vi "LV Demo Main.vi"() -> ()   [LabVIEW 2018, in "Powermeter_library.lvlib"]
uses:
  Powermeter_library.lvlib
  Channel States.ctl
  Global Variables.vi
  <vilib>/regexp/Match Regular Expression.xnode
panel:
  out "tdms error":errorcluster
  out "tdms file":refnum<k34>
  out "File Size (Mb)":dbl=76.0
  in  "Tab Control":enum32{"File", "Page 2"}(tab)
  out "file path":path=path "E:/Alkali metals/Excimer/2018-03-05/Run1_Powermeter.tdms"
  in  "Logfile?":bool=TRUE
  in  "Meas On":bool[](array[boolean])=[FALSE]
  in  "scan again":bool
  in  "All Handles":i32[](array[numeric])=[0]
  in  "Get Lib Ver":bool
  in  "Get Driver Ver":bool
  out "LibVer":i32
  out "DriverVer":string
  out "output cluster":T1
  in  "Reset graph 2":bool
  out "Timestamp offset":dbl
  out "First Data point":bool=TRUE
  out "Power meter 2":cluster{timestamp[], dbl[]}(graph)={[timestamp(3586444920.089349 s since 1904-01-01), timestamp(3586444920.2053604 s since 1904-01-01), timestamp(3586444920.2613664 s since 1904-01-01), timestamp(3586444920.370377 s since 1904-01-01), timestamp(3586444920.479388 s since 1904-01-01), timestamp(3586444920.588399 s since 1904-01-01), timestamp(3586444920.70241 s since 1904-01-01), timestamp(3586444920.7584157 s since 1904-01-01), timestamp(3586444920.868427 s since 1904-01-01), timestamp(3586444920.978438 s since 1904-01-01), timestamp(3586444921.0864487 s since 1904-01-01), timestamp(3586444921.19646 s since 1904-01-01), timestamp(3586444921.253465 s since 1904-01-01), timestamp(3586444921.3664765 s since 1904-01-01), timestamp(3586444921.6875086 s since 1904-01-01), timestamp(3586444921.7935195 s since 1904-01-01), timestamp(3586444922.0625463 s since 1904-01-01), timestamp(3586444922.170557 s since 1904-01-01), timestamp(3586444922.491589 s since 1904-01-01), timestamp(3586444922.6016 s since 1904-01-01), timestamp(3586444922.868627 s since 1904-01-01), timestamp(3586444922.977638 s since 1904-01-01), timestamp(3586444923.29867 s since 1904-01-01), timestamp(3586444923.3546753 s since 1904-01-01), timestamp(3586444923.6767077 s since 1904-01-01), timestamp(3586444923.7857184 s since 1904-01-01), timestamp(3586444924.0537453 s since 1904-01-01), timestamp(3586444924.161756 s since 1904-01-01), timestamp(3586444924.270767 s since 1904-01-01), timestamp(3586444924.379778 s since 1904-01-01), timestamp(3586444924.489789 s since 1904-01-01), timestamp(3586444924.6028004 s since 1904-01-01), timestamp(3586444924.6558056 s since 1904-01-01), timestamp(3586444924.772817 s since 1904-01-01), timestamp(3586444924.880828 s since 1904-01-01), timestamp(3586444924.952835 s since 1904-01-01), timestamp(3586444925.062846 s since 1904-01-01), timestamp(3586444925.168857 s since 1904-01-01), timestamp(3586444925.2788677 s since 1904-01-01), timestamp(3586444925.3868785 s since 1904-01-01), timestamp(3586444925.4968896 s since 1904-01-01), timestamp(3586444925.552895 s since 1904-01-01), timestamp(3586444925.6619062 s since 1904-01-01), timestamp(3586444925.770917 s since 1904-01-01), timestamp(3586444925.879928 s since 1904-01-01), timestamp(3586444925.987939 s since 1904-01-01), timestamp(3586444926.0939493 s since 1904-01-01), timestamp(3586444926.149955 s since 1904-01-01), timestamp(3586444926.2609663 s since 1904-01-01), timestamp(3586444926.370977 s since 1904-01-01), timestamp(3586444926.479988 s since 1904-01-01), timestamp(3586444926.588999 s since 1904-01-01), timestamp(3586444926.69801 s since 1904-01-01), timestamp(3586444926.7540154 s since 1904-01-01), timestamp(3586444926.863026 s since 1904-01-01), timestamp(3586444926.9760375 s since 1904-01-01), timestamp(3586444927.0850487 s since 1904-01-01), timestamp(3586444927.191059 s since 1904-01-01), timestamp(3586444927.30207 s since 1904-01-01), timestamp(3586444927.356076 s since 1904-01-01), timestamp(3586444927.4650865 s since 1904-01-01), timestamp(3586444927.5790977 s since 1904-01-01), timestamp(3586444927.688109 s since 1904-01-01), timestamp(3586444927.849125 s since 1904-01-01), timestamp(3586444927.9581356 s since 1904-01-01), timestamp(3586444928.0681467 s since 1904-01-01), timestamp(3586444928.180158 s since 1904-01-01), timestamp(3586444928.289169 s since 1904-01-01), timestamp(3586444928.39818 s since 1904-01-01), timestamp(3586444928.4661865 s since 1904-01-01), timestamp(3586444928.581198 s since 1904-01-01), timestamp(3586444928.6942096 s since 1904-01-01), timestamp(3586444928.750215 s since 1904-01-01), timestamp(3586444928.870227 s since 1904-01-01), timestamp(3586444928.9772377 s since 1904-01-01), timestamp(3586444929.0932493 s since 1904-01-01), timestamp(3586444929.149255 s since 1904-01-01), timestamp(3586444929.259266 s since 1904-01-01), timestamp(3586444929.3672767 s since 1904-01-01), timestamp(3586444929.4762874 s since 1904-01-01), timestamp(3586444929.5852985 s since 1904-01-01), timestamp(3586444929.694309 s since 1904-01-01), timestamp(3586444929.750315 s since 1904-01-01), timestamp(3586444929.862326 s since 1904-01-01), timestamp(3586444929.9763374 s since 1904-01-01), timestamp(3586444930.0863485 s since 1904-01-01), timestamp(3586444930.1943593 s since 1904-01-01), timestamp(3586444930.249365 s since 1904-01-01), timestamp(3586444930.358376 s since 1904-01-01), timestamp(3586444930.4763875 s since 1904-01-01), timestamp(3586444930.5853987 s since 1904-01-01), timestamp(3586444930.6944094 s since 1904-01-01), timestamp(3586444930.7514153 s since 1904-01-01), timestamp(3586444930.859426 s since 1904-01-01), timestamp(3586444930.9654365 s since 1904-01-01), timestamp(3586444931.0754476 s since 1904-01-01), timestamp(3586444931.190459 s since 1904-01-01), timestamp(3586444931.29947 s since 1904-01-01), timestamp(3586444931.3554754 s since 1904-01-01), timestamp(3586444931.4644866 s since 1904-01-01), timestamp(3586444931.7845182 s since 1904-01-01), timestamp(3586444931.8935294 s since 1904-01-01), timestamp(3586444931.949535 s since 1904-01-01), timestamp(3586444932.059546 s since 1904-01-01), timestamp(3586444932.1685567 s since 1904-01-01), timestamp(3586444932.277568 s since 1904-01-01), timestamp(3586444932.3875785 s since 1904-01-01), timestamp(3586444932.4965897 s since 1904-01-01), timestamp(3586444932.552595 s since 1904-01-01), timestamp(3586444932.6616063 s since 1904-01-01), timestamp(3586444932.770617 s since 1904-01-01), timestamp(3586444932.8796277 s since 1904-01-01), timestamp(3586444932.9866385 s since 1904-01-01), timestamp(3586444933.0956497 s since 1904-01-01), timestamp(3586444933.151655 s since 1904-01-01), timestamp(3586444933.2616663 s since 1904-01-01), timestamp(3586444933.374677 s since 1904-01-01), timestamp(3586444933.4836884 s since 1904-01-01), timestamp(3586444933.592699 s since 1904-01-01), timestamp(3586444933.649705 s since 1904-01-01), timestamp(3586444933.7587156 s since 1904-01-01), timestamp(3586444933.8667264 s since 1904-01-01), timestamp(3586444933.9757376 s since 1904-01-01), timestamp(3586444934.0837483 s since 1904-01-01), timestamp(3586444934.191759 s since 1904-01-01), timestamp(3586444934.29977 s since 1904-01-01), timestamp(3586444934.3557754 s since 1904-01-01), timestamp(3586444934.4647865 s since 1904-01-01), timestamp(3586444934.573797 s since 1904-01-01), timestamp(3586444934.6828084 s since 1904-01-01), timestamp(3586444934.791819 s since 1904-01-01), timestamp(3586444934.89883 s since 1904-01-01), timestamp(3586444934.9548354 s since 1904-01-01), timestamp(3586444935.063846 s since 1904-01-01), timestamp(3586444935.171857 s since 1904-01-01), timestamp(3586444935.280868 s since 1904-01-01), timestamp(3586444935.3898787 s since 1904-01-01), timestamp(3586444935.49989 s since 1904-01-01), timestamp(3586444935.5568957 s since 1904-01-01), timestamp(3586444935.6659064 s since 1904-01-01), timestamp(3586444935.770917 s since 1904-01-01), timestamp(3586444935.879928 s since 1904-01-01), timestamp(3586444935.988939 s since 1904-01-01), timestamp(3586444936.0979495 s since 1904-01-01), timestamp(3586444936.1539555 s since 1904-01-01), timestamp(3586444936.261966 s since 1904-01-01), timestamp(3586444936.370977 s since 1904-01-01), timestamp(3586444936.479988 s since 1904-01-01), timestamp(3586444936.588999 s since 1904-01-01), timestamp(3586444936.69901 s since 1904-01-01), timestamp(3586444936.7550154 s since 1904-01-01), timestamp(3586444936.864026 s since 1904-01-01), timestamp(3586444936.9720373 s since 1904-01-01), timestamp(3586444937.081048 s since 1904-01-01), timestamp(3586444937.189059 s since 1904-01-01), timestamp(3586444937.29907 s since 1904-01-01), timestamp(3586444937.3550754 s since 1904-01-01), timestamp(3586444937.4640865 s since 1904-01-01), timestamp(3586444937.573097 s since 1904-01-01), timestamp(3586444937.6831083 s since 1904-01-01)], [0.0, 0.0, 0.0, 0.0, 0.0, 0.0, 0.0, 0.0, 0.0, 0.0, 0.0, 0.0, 0.0, 0.0, 0.0, 0.0, 0.0, 0.0, 0.0, 0.0, 0.0, 0.0, 0.0, 0.0, 0.0, 0.0, 0.0, 0.0, 0.0, 0.0, 0.0, 0.0, 0.0, 0.0, 0.0, 0.0, 0.0, 0.0, 0.0, 0.0, 0.0, 0.0, 0.0, 0.0, 0.0, 0.0, 0.0, 0.0, 0.0, 0.0, 0.0, 0.0, 0.0, 0.0, 0.0, 0.0, 0.0, 0.0, 0.0, 0.0, 0.0, 0.0, 0.0, 0.0, 0.0, 0.0, 0.0, 0.0, 0.0, 0.0, 0.0, 0.0, 0.0, 0.0, 0.0, 0.0, 0.0, 0.0, 0.0, 0.0, 0.0, 0.0, 0.0, 0.0, 0.0, 0.0, 0.0, 0.0, 0.0, 0.0, 0.0, 0.0, 0.0, 0.0, 0.0, 0.0, 0.0, 0.0, 0.0, 0.0, 0.0, 0.0, 0.0, 0.0, 0.0, 0.0, 0.0, 0.0, 0.0, 0.0, 0.0, 0.0, 0.0, 0.0, 0.0, 0.0, 0.0, 0.0, 0.0, 0.0, 0.0, 0.0, 0.0, 0.0, 0.0, 0.0, 0.0, 0.0, 0.0, 0.0, 0.0, 0.0, 0.0, 0.0, 0.0, 0.0, 0.0, 0.0, 0.0, 0.0, 0.0, 0.0, 0.0, 0.0, 0.0, 0.0, 0.0, 0.0, 0.0, 0.0, 0.0, 0.0, 0.0, 0.0, 0.0, 0.0, 0.0, 0.0, 0.0, 0.0]}
  in  "Reset graph 1":bool
  out "Power meter 1":cluster{timestamp[], dbl[]}(graph)={[timestamp(3586444920.089349 s since 1904-01-01), timestamp(3586444920.2053604 s since 1904-01-01), timestamp(3586444920.2613664 s since 1904-01-01), timestamp(3586444920.370377 s since 1904-01-01), timestamp(3586444920.479388 s since 1904-01-01), timestamp(3586444920.588399 s since 1904-01-01), timestamp(3586444920.70241 s since 1904-01-01), timestamp(3586444920.7584157 s since 1904-01-01), timestamp(3586444920.868427 s since 1904-01-01), timestamp(3586444920.978438 s since 1904-01-01), timestamp(3586444921.0864487 s since 1904-01-01), timestamp(3586444921.19646 s since 1904-01-01), timestamp(3586444921.253465 s since 1904-01-01), timestamp(3586444921.3664765 s since 1904-01-01), timestamp(3586444921.6875086 s since 1904-01-01), timestamp(3586444921.7935195 s since 1904-01-01), timestamp(3586444922.0625463 s since 1904-01-01), timestamp(3586444922.170557 s since 1904-01-01), timestamp(3586444922.491589 s since 1904-01-01), timestamp(3586444922.6016 s since 1904-01-01), timestamp(3586444922.868627 s since 1904-01-01), timestamp(3586444922.977638 s since 1904-01-01), timestamp(3586444923.29867 s since 1904-01-01), timestamp(3586444923.3546753 s since 1904-01-01), timestamp(3586444923.6767077 s since 1904-01-01), timestamp(3586444923.7857184 s since 1904-01-01), timestamp(3586444924.0537453 s since 1904-01-01), timestamp(3586444924.161756 s since 1904-01-01), timestamp(3586444924.270767 s since 1904-01-01), timestamp(3586444924.379778 s since 1904-01-01), timestamp(3586444924.489789 s since 1904-01-01), timestamp(3586444924.6028004 s since 1904-01-01), timestamp(3586444924.6558056 s since 1904-01-01), timestamp(3586444924.772817 s since 1904-01-01), timestamp(3586444924.880828 s since 1904-01-01), timestamp(3586444924.952835 s since 1904-01-01), timestamp(3586444925.062846 s since 1904-01-01), timestamp(3586444925.168857 s since 1904-01-01), timestamp(3586444925.2788677 s since 1904-01-01), timestamp(3586444925.3868785 s since 1904-01-01), timestamp(3586444925.4968896 s since 1904-01-01), timestamp(3586444925.552895 s since 1904-01-01), timestamp(3586444925.6619062 s since 1904-01-01), timestamp(3586444925.770917 s since 1904-01-01), timestamp(3586444925.879928 s since 1904-01-01), timestamp(3586444925.987939 s since 1904-01-01), timestamp(3586444926.0939493 s since 1904-01-01), timestamp(3586444926.149955 s since 1904-01-01), timestamp(3586444926.2609663 s since 1904-01-01), timestamp(3586444926.370977 s since 1904-01-01), timestamp(3586444926.479988 s since 1904-01-01), timestamp(3586444926.588999 s since 1904-01-01), timestamp(3586444926.69801 s since 1904-01-01), timestamp(3586444926.7540154 s since 1904-01-01), timestamp(3586444926.863026 s since 1904-01-01), timestamp(3586444926.9760375 s since 1904-01-01), timestamp(3586444927.0850487 s since 1904-01-01), timestamp(3586444927.191059 s since 1904-01-01), timestamp(3586444927.30207 s since 1904-01-01), timestamp(3586444927.356076 s since 1904-01-01), timestamp(3586444927.4650865 s since 1904-01-01), timestamp(3586444927.5790977 s since 1904-01-01), timestamp(3586444927.688109 s since 1904-01-01), timestamp(3586444927.849125 s since 1904-01-01), timestamp(3586444927.9581356 s since 1904-01-01), timestamp(3586444928.0681467 s since 1904-01-01), timestamp(3586444928.180158 s since 1904-01-01), timestamp(3586444928.289169 s since 1904-01-01), timestamp(3586444928.39818 s since 1904-01-01), timestamp(3586444928.4661865 s since 1904-01-01), timestamp(3586444928.581198 s since 1904-01-01), timestamp(3586444928.6942096 s since 1904-01-01), timestamp(3586444928.750215 s since 1904-01-01), timestamp(3586444928.870227 s since 1904-01-01), timestamp(3586444928.9772377 s since 1904-01-01), timestamp(3586444929.0932493 s since 1904-01-01), timestamp(3586444929.149255 s since 1904-01-01), timestamp(3586444929.259266 s since 1904-01-01), timestamp(3586444929.3672767 s since 1904-01-01), timestamp(3586444929.4762874 s since 1904-01-01), timestamp(3586444929.5852985 s since 1904-01-01), timestamp(3586444929.694309 s since 1904-01-01), timestamp(3586444929.750315 s since 1904-01-01), timestamp(3586444929.862326 s since 1904-01-01), timestamp(3586444929.9763374 s since 1904-01-01), timestamp(3586444930.0863485 s since 1904-01-01), timestamp(3586444930.1943593 s since 1904-01-01), timestamp(3586444930.249365 s since 1904-01-01), timestamp(3586444930.358376 s since 1904-01-01), timestamp(3586444930.4763875 s since 1904-01-01), timestamp(3586444930.5853987 s since 1904-01-01), timestamp(3586444930.6944094 s since 1904-01-01), timestamp(3586444930.7514153 s since 1904-01-01), timestamp(3586444930.859426 s since 1904-01-01), timestamp(3586444930.9654365 s since 1904-01-01), timestamp(3586444931.0754476 s since 1904-01-01), timestamp(3586444931.190459 s since 1904-01-01), timestamp(3586444931.29947 s since 1904-01-01), timestamp(3586444931.3554754 s since 1904-01-01), timestamp(3586444931.4644866 s since 1904-01-01), timestamp(3586444931.7845182 s since 1904-01-01), timestamp(3586444931.8935294 s since 1904-01-01), timestamp(3586444931.949535 s since 1904-01-01), timestamp(3586444932.059546 s since 1904-01-01), timestamp(3586444932.1685567 s since 1904-01-01), timestamp(3586444932.277568 s since 1904-01-01), timestamp(3586444932.3875785 s since 1904-01-01), timestamp(3586444932.4965897 s since 1904-01-01), timestamp(3586444932.552595 s since 1904-01-01), timestamp(3586444932.6616063 s since 1904-01-01), timestamp(3586444932.770617 s since 1904-01-01), timestamp(3586444932.8796277 s since 1904-01-01), timestamp(3586444932.9866385 s since 1904-01-01), timestamp(3586444933.0956497 s since 1904-01-01), timestamp(3586444933.151655 s since 1904-01-01), timestamp(3586444933.2616663 s since 1904-01-01), timestamp(3586444933.374677 s since 1904-01-01), timestamp(3586444933.4836884 s since 1904-01-01), timestamp(3586444933.592699 s since 1904-01-01), timestamp(3586444933.649705 s since 1904-01-01), timestamp(3586444933.7587156 s since 1904-01-01), timestamp(3586444933.8667264 s since 1904-01-01), timestamp(3586444933.9757376 s since 1904-01-01), timestamp(3586444934.0837483 s since 1904-01-01), timestamp(3586444934.191759 s since 1904-01-01), timestamp(3586444934.29977 s since 1904-01-01), timestamp(3586444934.3557754 s since 1904-01-01), timestamp(3586444934.4647865 s since 1904-01-01), timestamp(3586444934.573797 s since 1904-01-01), timestamp(3586444934.6828084 s since 1904-01-01), timestamp(3586444934.791819 s since 1904-01-01), timestamp(3586444934.89883 s since 1904-01-01), timestamp(3586444934.9548354 s since 1904-01-01), timestamp(3586444935.063846 s since 1904-01-01), timestamp(3586444935.171857 s since 1904-01-01), timestamp(3586444935.280868 s since 1904-01-01), timestamp(3586444935.3898787 s since 1904-01-01), timestamp(3586444935.49989 s since 1904-01-01), timestamp(3586444935.5568957 s since 1904-01-01), timestamp(3586444935.6659064 s since 1904-01-01), timestamp(3586444935.770917 s since 1904-01-01), timestamp(3586444935.879928 s since 1904-01-01), timestamp(3586444935.988939 s since 1904-01-01), timestamp(3586444936.0979495 s since 1904-01-01), timestamp(3586444936.1539555 s since 1904-01-01), timestamp(3586444936.261966 s since 1904-01-01), timestamp(3586444936.370977 s since 1904-01-01), timestamp(3586444936.479988 s since 1904-01-01), timestamp(3586444936.588999 s since 1904-01-01), timestamp(3586444936.69901 s since 1904-01-01), timestamp(3586444936.7550154 s since 1904-01-01), timestamp(3586444936.864026 s since 1904-01-01), timestamp(3586444936.9720373 s since 1904-01-01), timestamp(3586444937.081048 s since 1904-01-01), timestamp(3586444937.189059 s since 1904-01-01), timestamp(3586444937.29907 s since 1904-01-01), timestamp(3586444937.3550754 s since 1904-01-01), timestamp(3586444937.4640865 s since 1904-01-01), timestamp(3586444937.573097 s since 1904-01-01), timestamp(3586444937.6831083 s since 1904-01-01)], [0.0, 0.0, 0.0, 0.0, 0.0, 0.0, 0.0, 0.0, 0.0, 0.0, 0.0, 0.0, 0.0, 0.0, 0.0, 0.0, 0.0, 0.0, 0.0, 0.0, 0.0, 0.0, 0.0, 0.0, 0.0, 0.0, 0.0, 0.0, 0.0, 0.0, 0.0, 0.0, 0.0, 0.0, 0.0, 0.0, 0.0, 0.0, 0.0, 0.0, 0.0, 0.0, 0.0, 0.0, 0.0, 0.0, 0.0, 0.0, 0.0, 0.0, 0.0, 0.0, 0.0, 0.0, 0.0, 0.0, 0.0, 0.0, 0.0, 0.0, 0.0, 0.0, 0.0, 0.0, 0.0, 0.0, 0.0, 0.0, 0.0, 0.0, 0.0, 0.0, 0.0, 0.0, 0.0, 0.0, 0.0, 0.0, 0.0, 0.0, 0.0, 0.0, 0.0, 0.0, 0.0, 0.0, 0.0, 0.0, 0.0, 0.0, 0.0, 0.0, 0.0, 0.0, 0.0, 0.0, 0.0, 0.0, 0.0, 0.0, 0.0, 0.0, 0.0, 0.0, 0.0, 0.0, 0.0, 0.0, 0.0, 0.0, 0.0, 0.0, 0.0, 0.0, 0.0, 0.0, 0.0, 0.0, 0.0, 0.0, 0.0, 0.0, 0.0, 0.0, 0.0, 0.0, 0.0, 0.0, 0.0, 0.0, 0.0, 0.0, 0.0, 0.0, 0.0, 0.0, 0.0, 0.0, 0.0, 0.0, 0.0, 0.0, 0.0, 0.0, 0.0, 0.0, 0.0, 0.0, 0.0, 0.0, 0.0, 0.0, 0.0, 0.0, 0.0, 0.0, 0.0, 0.0, 0.0, 0.0]}
  in  "Save data":bool=TRUE
  in  "Stop":bool
  out "ReadStr":string
  in  "Read/Write":T2
  out "Device Name":string="(0)"
  in  "Dev Control":T3 {"externTrigModes" items=["Rising Edge", "Falling Edge", "High Level", "Low Level", "Output High", "Output Low"]; "Stream Modes:" items=["Turbo", "Turbo Freq", "Immediate"]}
  out "Last Error Code:":string
  in  "Gen'l Ops":T4
  # "Local variables"
  # "v1.14"
  # "Write / Read"
  # "Device Control"
  # "Streams:"
  # "Ext Trig::"
  # "Device Management"
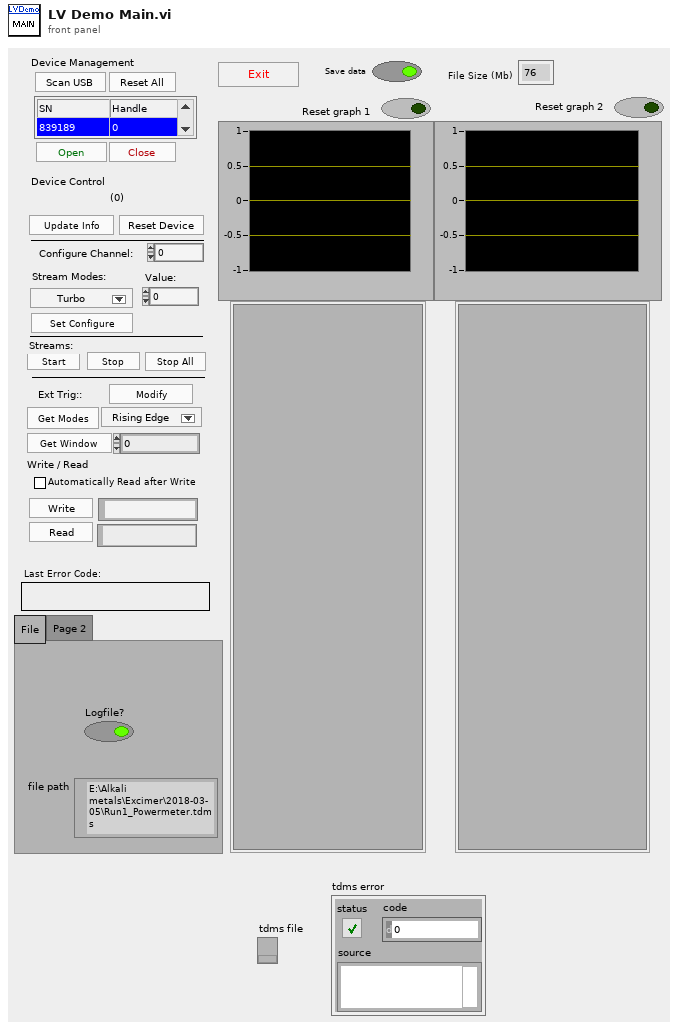
[diagram p1: front panel]
types:
  T1 = cluster{"output cluster 2":cluster{"Value:":dbl[], timestamp[], string[][]}, "output cluster 3":cluster{"Value:":dbl[], timestamp[], string[][]}}
  T2 = cluster{"AutoRead":bool, "Write":bool, "Read":bool, "WriteStr":string}
  T3 = cluster{"UpdateInfo":bool, "ResetDev":bool, "ConfigCh":i32, "Stream Modes:":i32, "Value":i32, "SetConfig":bool, "StartStream":bool, "StopStream":bool, "StopAll":bool, "externTrigModes":i32, "GetModes":bool, "GetWindow":bool, "ExtTrig Window":i32, "Modify":bool}
  T4 = cluster{"scanUSB":bool, "Devices":i32, "Open":bool, "Close":bool, "ResetAll":bool}
  T5 = enum16{"open", "open or create", "create or replace", "create", "open (read-only)"}
  T6 = typedef "Powermeter_library.lvlib/Channel States.ctl" = enum16{"Init", "Poll", "Set Handle", "Measure"}
  T7 = cluster{"Value:":dbl[], " Time:":string[], " Status:":string[]}
  T8 = enum32{"invalid app kind", "Development System", "Run Time System", "Student Edition", "Embedded LabVIEW", "Evaluation", "Custom"}
  T9 = cluster{"Project":u16, "SubFolder":string, "Filename (Meas. Description)":string, "Measurement index":i32}
  T10 = cluster{"Value:":dbl[], " Time:":string[], " Status:":string[]}[]
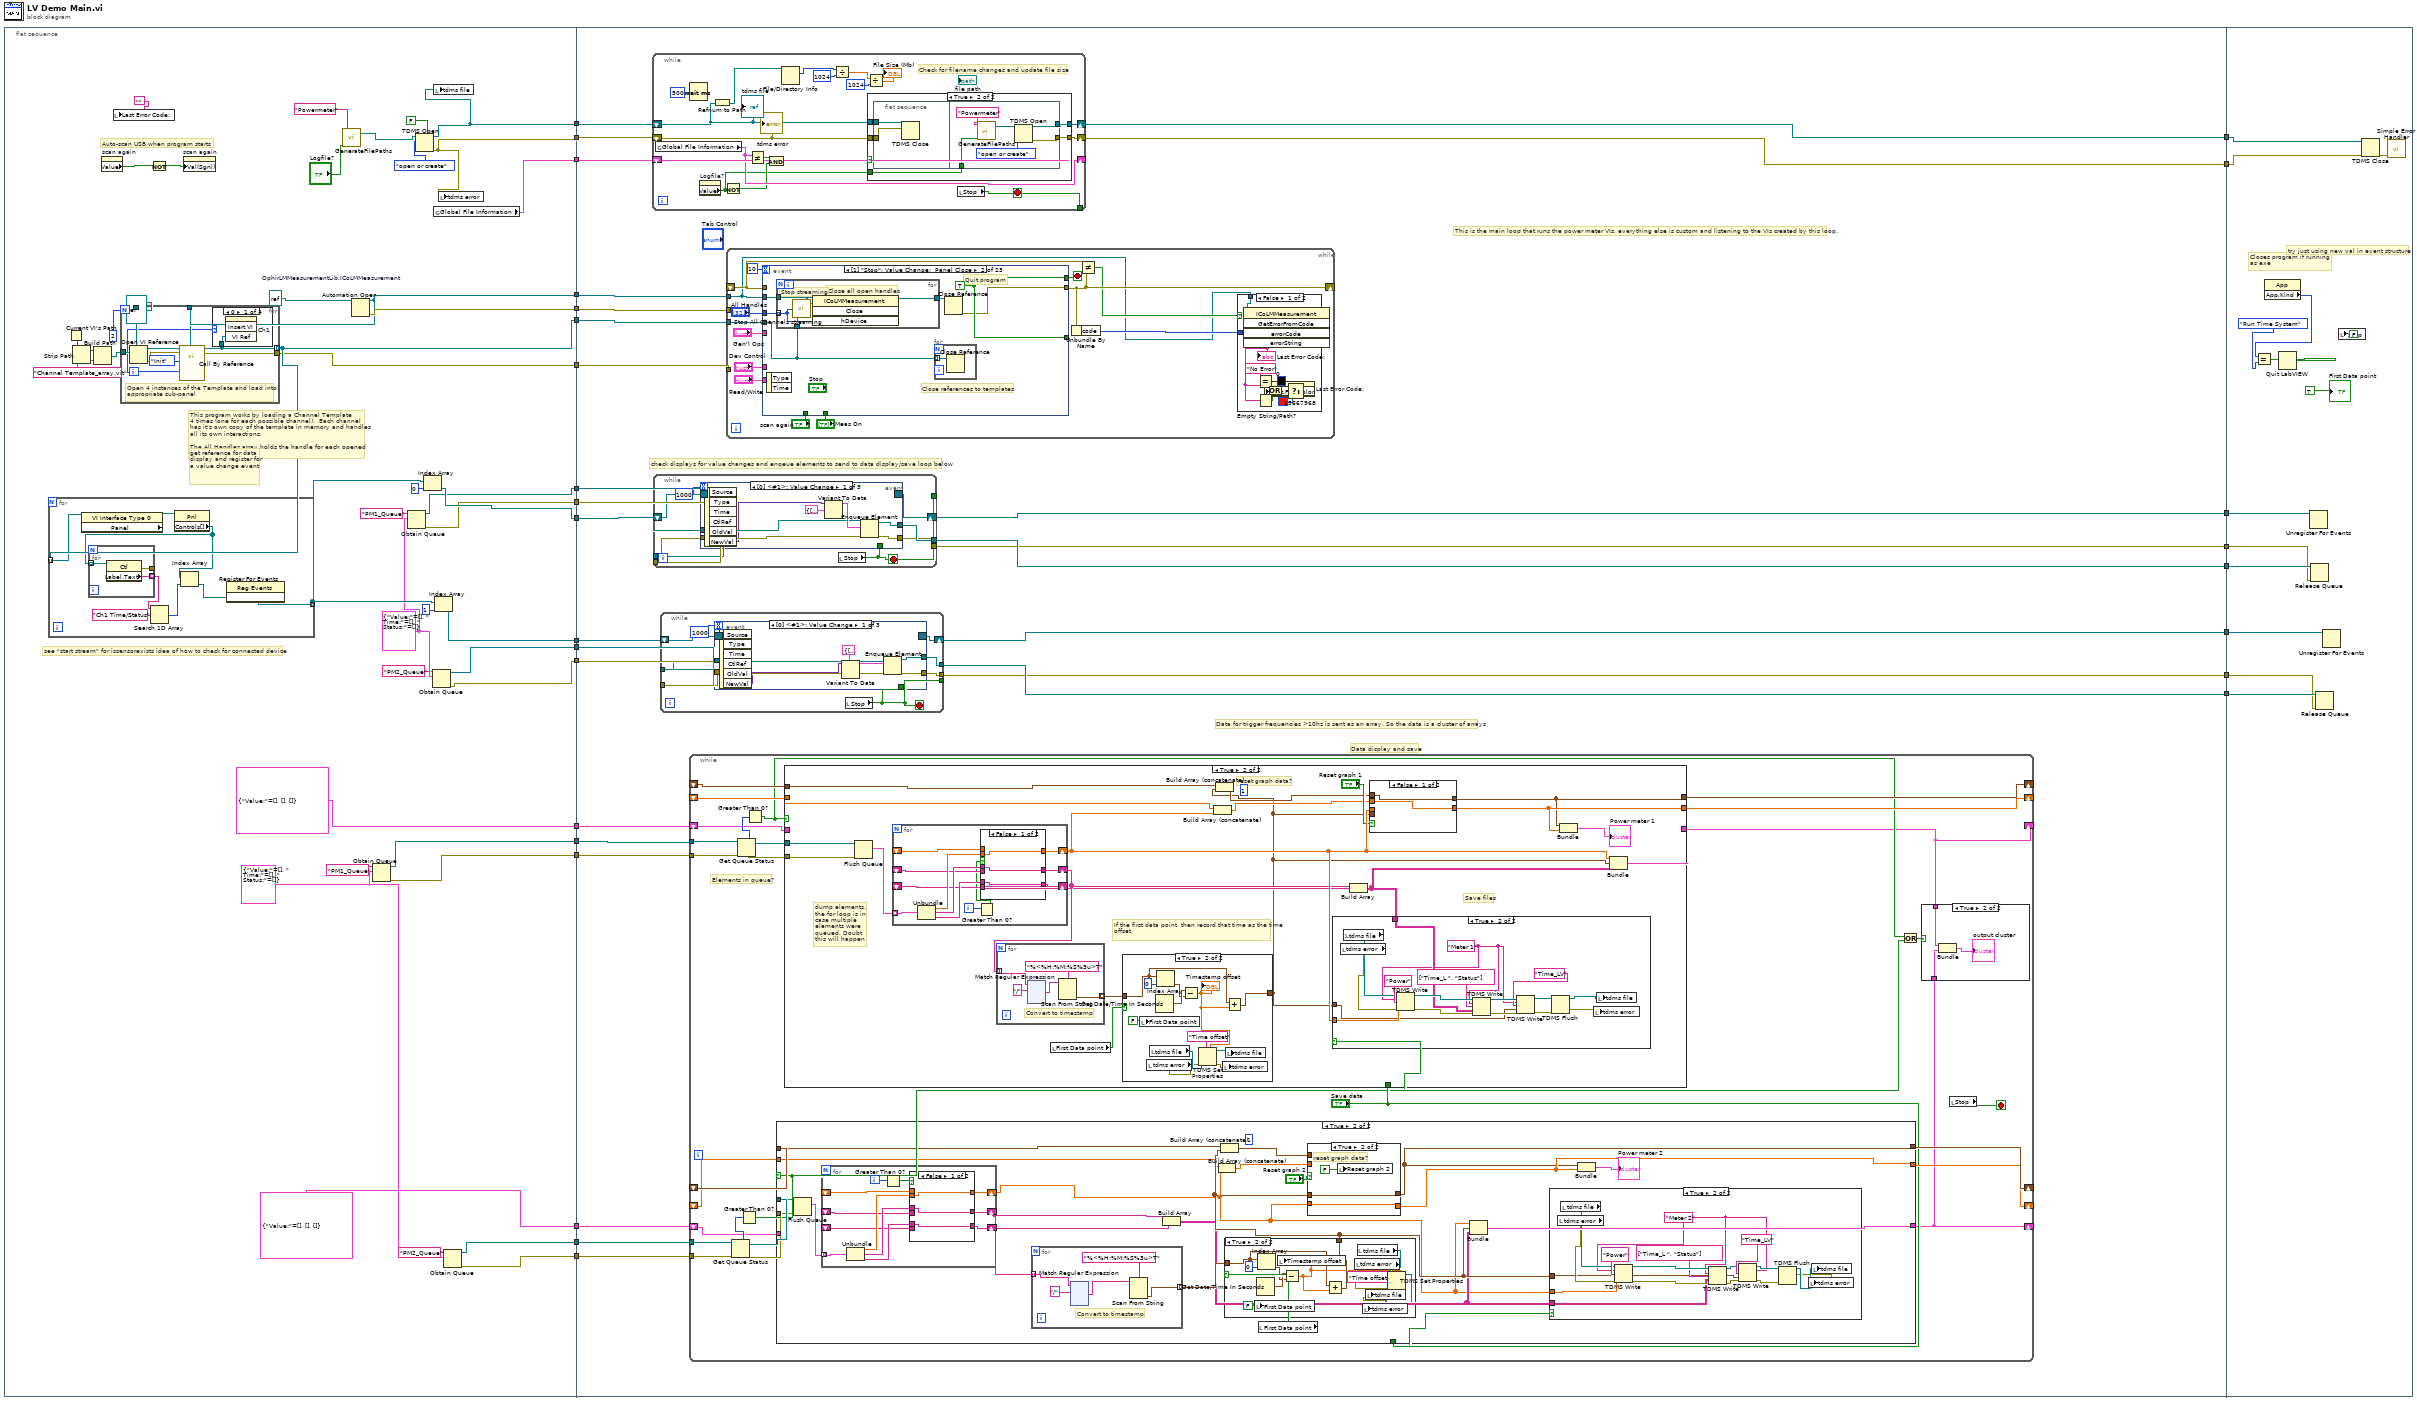
[diagram p0: block diagram]
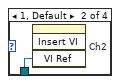
[diagram p2: hidden frame]
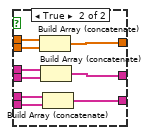
[diagram p6: hidden frame]
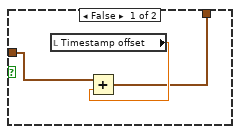
[diagram p8: hidden frame]
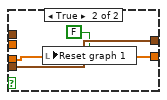
[diagram p11: hidden frame]
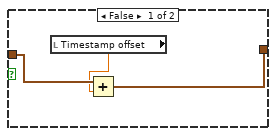
[diagram p12: hidden frame]
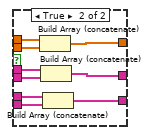
[diagram p14: hidden frame]
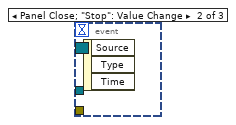
[diagram p16: hidden frame]
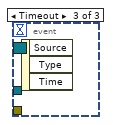
[diagram p17: hidden frame]
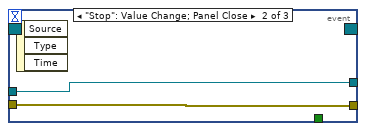
[diagram p18: hidden frame]
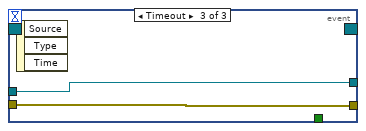
[diagram p19: hidden frame]
diagram:
  n1 = flat-sequence {
    tunnel: [w30] -> w25
    tunnel: [w47] -> w24
    tunnel: [w48] -> w23
    tunnel: [w35] -> w22
    tunnel: [w34] -> w21
    tunnel: [w31] -> w20
    tunnel: [w36] -> w19
    tunnel: [w32] -> w18
    tunnel: [w37] -> w17
    tunnel: [w33] -> w16
    tunnel: [w40] -> w15
    tunnel: [w41] -> w14
    tunnel: [w39] -> w13
    tunnel: [w38] -> w12
    tunnel: [cluster{"Value:":dbl[], timestamp[], string[][]} {"Value:"=[], [], []} ("output cluster 3")] -> w11
    tunnel: [cluster{"Value:":dbl[], timestamp[], string[][]} {"Value:"=[], [], []} ("output cluster 2")] -> w10
    tunnel: [w44] -> w9
    tunnel: [w45] -> w8
    tunnel: [w46] -> w7
    tunnel: [w102] -> w27
    tunnel: [w101] -> w26
    tunnel: w25 -> [w119]
    tunnel: w24 -> [w118]
    tunnel: w23 -> [w117]
    tunnel: w22 -> [w116]
    tunnel: w21 -> [w115]
    tunnel: w20 -> [w114]
    tunnel: w19 -> [w113]
    tunnel: w18 -> [w112]
    tunnel: w17 -> [w111]
    tunnel: w16 -> [w110]
    tunnel: w15 -> [w109]
    tunnel: w14 -> [w108]
    tunnel: w13 -> [w107]
    tunnel: w12 -> [w106]
    tunnel: w11 -> [w105]
    tunnel: w10 -> [w104]
    tunnel: w9 -> [w103]
    tunnel: w8 -> [w100]
    tunnel: w7 -> [w99]
    tunnel: [w98] -> w6
    tunnel: [w97] -> w5
    tunnel: [w96] -> w4
    tunnel: [w95] -> w3
    tunnel: [w94] -> w2
    tunnel: [w93] -> w1
    tunnel: w27 -> [w926]
    tunnel: w26 -> [w927]
    tunnel: w6 -> [w923]
    tunnel: w5 -> [w922]
    tunnel: w4 -> [w921]
    tunnel: w3 -> [w920]
    tunnel: w2 -> [w919]
    tunnel: w1 -> [w918]
    frame #0 {
      w56 = T7 {"Value:"=[], " Time:"=[], " Status:"=[]} ("Ch1 Time/Status")
      w54 = T7 {"Value:"=[], " Time:"=[], " Status:"=[]} ("Ch1 Time/Status")
      w64 = refnum<k7> refnum  # OphirLMMeasurementLib.ICoLMMeasurement
      # "get reference for data display and register for a value change event"
      # "see \"start stream\" for issensorexists idea of how to check for connected device"
      # "This program works by loading a Channel Template\n4 times (one for each possible channel).  Each channel\nhas it's own copy of the template in memory and handles\nall its own interactions. \n\nThe All Handles array holds the handle for each opened device"
      # "Auto-scan USB when program starts"
      n2 = Current VI's Path() -> (path=w65:path)
      n3 = Strip Path(path=w65) -> (stripped path=w66:path)  [unwired: 1 out]
      n4 = Build Path(base path=w66, name or relative path="Channel Template_array.vit") -> (appended path=w67:path)
      n5 = property on="scan again" class="Bool (strict)"() -> ("Value"=w69:bool)  [unwired: 2 in, 2 out]
      n6 = local write "Last Error Code:"("") -> ()
      n7 = Not(x=w69) -> (.not. x?=w68:bool)
      n8 = property on="scan again" class="Bool (strict)"("Val(Sgnl)"=w68) -> ()  [unwired: 2 in, 2 out]
      n9 = call "GenerateFilePaths.vi"("Logfile?"="Logfile?", "Device Name"="Powermeter") -> ("Path"=w28:path)  [unwired: 3 in]
      n10 = Automation Open(Automation Refnum=w64) -> (Automation Refnum=w47:refnum<k7>, error out=w48:errorcluster)  [unwired: 1 in, 2 out]
      n11 = for {
        N: 2 -> [_]
        tunnel: w67 -> [w90]
        tunnel: refnum<vi> refnum ("type specifier VI Refnum (for type only)") -> [w89]
        tunnel: w47 -> [w86]
        tunnel: [w82] -> w31 mode=indexing
        tunnel: [w84] -> w30
        i -> [w83]
        # "Open 4 instances of the Template and load into\nappropriate sub-panel"
        n12 = Open VI Reference(type specifier VI Refnum (for type only)=w89, vi path=w90) -> (vi reference=w88:refnum<vi>, error out=w85:errorcluster)  [unwired: 1 in, 3 out]
        n13 = call-by-ref "?"(reference=w88, error in=w85, "OphirLMMeasurementLib.ICoLMMeasurement"=w86, "Ch in"=w83, "State"=Channel_States."Init") -> (reference out=w82:refnum<vi>, error out=w84:errorcluster)  [unwired: 7 in, 1 out]
        n14 = case shown="0" w83 {
          tunnel: w82 -> [w91 w92 _ _]
          frame 0 {
            n15 = invoke on="Ch1" class="SubPnl" method="Insert VI"("VI Ref"=w91) -> ()  [unwired: 3 in, 4 out]
          }
          frame 1, Default {
            n16 = invoke on="Ch2" class="SubPnl" method="Insert VI"("VI Ref"=w92) -> ()  [unwired: 3 in, 4 out]
          }
          frame 2 {
          }
          frame 3 {
          }
        }
      }
      n17 = for {
        tunnel: w31 -> [w77] mode=indexing
        tunnel: [w71] -> w70 mode=indexing
        n18 = property class="VI Interface Type 0"(reference=w77) -> ("Panel"=w78:refnum<vi>)  [unwired: 1 in, 2 out]
        n19 = property class="Pnl"(reference=w78) -> ("Controls[]"=w74:refnum<vi>[])  [unwired: 1 in, 2 out]
        n20 = for {
          tunnel: w74 -> [w81] mode=indexing
          tunnel: [w80] -> w76 mode=indexing
          tunnel: [w79] -> _
          n21 = property class="Ctl"(reference=w81) -> (error out=w79:errorcluster, "Label.Text"=w80:string)  [unwired: 1 in, 1 out]
        }
        n22 = Search 1D Array(1D array=w76, element="Ch1 Time/Status") -> (index of element=w73:i32)  [unwired: 1 in]
        n23 = Index Array(array=w74, index=w73) -> (element=w72:refnum<vi>)
        n24 = register-events(w72) -> (reference out=w71:refnum<event-registration>)  [unwired: 2 in, 1 out]
      }
      n25 = Obtain Queue(name (unnamed)="PM1_Queue", element data type=w56) -> (queue out=w35:refnum<queue>, error out=w34:errorcluster)  [unwired: 3 in, 1 out]
      n26 = Obtain Queue(name (unnamed)="PM1_Queue", element data type=w54) -> (queue out=w37:refnum<queue>, error out=w36:errorcluster)  [unwired: 3 in, 1 out]
      n27 = TDMS Open(5:FALSE ("create index file? (T)"), 10:T5."open or create" ("operation (0:open)"), 11:w28) -> (0:w46:errorcluster, 3:w45:refnum<k34>)  [unwired: 4 in]
      n28 = Index Array(array=w70, index=0) -> (element=w40:refnum<event-registration>)
      n29 = Obtain Queue(name (unnamed)="PM2_Queue", element data type=w54) -> (queue out=w33:refnum<queue>, error out=w32:errorcluster)  [unwired: 3 in, 1 out]
      n30 = local write "tdms file"(w45) -> ()
      n31 = global read "Global Variables.vi" "Global File Information"() -> (w44:T9)
      n32 = Index Array(array=w70, index=1) -> (element=w41:refnum<event-registration>)
      n33 = local write "tdms error"(w46) -> ()
      n34 = Obtain Queue(name (unnamed)="PM2_Queue", element data type=w56) -> (queue out=w39:refnum<queue>, error out=w38:errorcluster)  [unwired: 3 in, 1 out]
    }
    frame #1 {
      # "This is the main loop that runs the power meter VIs, everything else is custom and listening to the VIs created by this loop."
      # "Data for trigger frequencies >10hz is sent as an array. So the data is a cluster of arrays"
      # "Data display and save"
      # "check displays for value changes and enqeue elements to send to data display/save loop below"
      n35 = while {
        tunnel: [w902] -> _
        shift-right: [w900] -> w102
        shift-left: w100 -> [w896]
        shift-right: [w899] -> w101
        shift-left: w99 -> [w901]
        shift-right: [w897] -> _
        shift-left: w103 -> [w898]
        stop <- w902 stop-if-true
        # "Check for filename changes and update file size"
        n36 = global read "Global Variables.vi" "Global File Information"() -> (w897:T9)
        n37 = Wait (ms)(milliseconds to wait=500) -> ()  [unwired: 1 out]
        n38 = property on="Logfile?" class="Bool (strict)"() -> ("Value"=w890:bool)  [unwired: 2 in, 2 out]
        n39 = Refnum to Path(1:w896) -> (0:w894:path)
        n40 = Not(x=w890) -> (.not. x?=w891:bool)
        n41 = Not Equal?(x=w897, y=w898) -> (x != y?=w893:bool)
        n42 = And(x=w893, y=w891) -> (x .and. y?=w892:bool)
        n43 = File/Directory Info(path=w894) -> (size=w886:i64)  [unwired: 1 in, 6 out]
        n44 = Divide(x=w886, y=i64 1024) -> (x/y=w887:dbl)
        n45 = Divide(x=w887, y=i64 1024) -> (x/y=→"File Size (Mb)":dbl)
        n46 = case shown="True" w892 {
          tunnel: w896 -> [w904 w909]
          tunnel: w901 -> [w903 w908]
          tunnel: [w904 w907] -> w900
          tunnel: [w903 w906] -> w899
          tunnel: w890 -> [_ w905]
          frame False {
          }
          frame True {
            n47 = flat-sequence {
              tunnel: w909 -> [w911]
              tunnel: w908 -> [w910]
              tunnel: [w917] -> w907
              tunnel: [w916] -> w906
              tunnel: w905 -> [w912]
              frame #0 {
                n48 = TDMS Close(8:w910, 11:w911) -> ()  [unwired: 2 out]
              }
              frame #1 {
                n49 = call "GenerateFilePaths.vi"("Logfile?"=w912, "Device Name"="Powermeter") -> ("Path"=w914:path)  [unwired: 3 in]
                n50 = TDMS Open(10:T5."open or create" ("operation (0:open)"), 11:w914) -> (0:w916:errorcluster, 3:w917:refnum<k34>)  [unwired: 5 in]
              }
            }
          }
        }
        n51 = local read "Stop"() -> (w902:bool)
        "tdms file" <- w896
        "tdms error" <- w901
      }
      n52 = while {
        shift-right: [w575] -> w97
        shift-left: w109 -> [w573]
        tunnel: [w572] -> _
        tunnel: w111 -> [w574]
        tunnel: [w577] -> w96
        tunnel: w113 -> [w578]
        tunnel: [w576] -> w95
        stop <- w572 stop-if-true
        n53 = local read "Stop"() -> (w572:bool)
        n54 = event shown="[0] <#1>: Value Change" {
          selector: w573 -> [_ _ _]
          dyn-events: [_ _ _] -> w575
          timeout: 1000 -> [_ _ _]
          tunnel: w574 -> [w583 w587 w589]
          tunnel: w578 -> [w582 w586 w588]
          tunnel: [w581 w587 w589] -> w577
          tunnel: [w580 w586 w588] -> w576
          tunnel: w572 -> [_ _ _]
          event Value Change {
            n55 = event-data() -> ("NewVal"=w579:variant)  [unwired: 1 in, 5 out]
            n56 = Variant To Data(type=T7 {"Value:"=[], " Time:"=[], " Status:"=[]} ("Ch1 Time/Status"), Variant=w579) -> (data=w584:T7)  [unwired: 1 in, 1 out]
            n57 = Enqueue Element(queue=w583, element=w584, error in (no error)=w582) -> (queue out=w581:refnum<queue>, error out=w580:errorcluster)  [unwired: 1 in, 1 out]
          }
          event "Stop": Value Change; Panel Close {
            n58 = event-data() -> ()  [unwired: 1 in, 3 out]
          }
          event Timeout {
            n59 = event-data() -> ()  [unwired: 1 in, 3 out]
          }
        }
      }
      n60 = while {
        shift-right: [w560] -> w98
        shift-left: w108 -> [w558]
        tunnel: [w557] -> _
        tunnel: w110 -> [w559]
        tunnel: [w562] -> w94
        tunnel: w112 -> [w563]
        tunnel: [w561] -> w93
        stop <- w557 stop-if-true
        n61 = local read "Stop"() -> (w557:bool)
        n62 = event shown="[0] <#1>: Value Change" {
          selector: w558 -> [_ _ _]
          dyn-events: [_ _ _] -> w560
          timeout: 1000 -> [_ _ _]
          tunnel: w563 -> [w569 _ _]
          tunnel: w559 -> [w567 _ _]
          tunnel: [w566 _ _] -> w562
          tunnel: [w565 _ _] -> w561
          tunnel: w557 -> [_ _ _]
          event Value Change {
            n63 = event-data() -> ("NewVal"=w564:variant)  [unwired: 1 in, 5 out]
            n64 = Variant To Data(type=T7 {"Value:"=[], " Time:"=[], " Status:"=[]} ("Ch1 Time/Status"), Variant=w564) -> (data=w568:T7)  [unwired: 1 in, 1 out]
            n65 = Enqueue Element(queue=w567, element=w568, error in (no error)=w569) -> (queue out=w566:refnum<queue>, error out=w565:errorcluster)  [unwired: 1 in, 1 out]
          }
          event Panel Close; "Stop": Value Change {
            n66 = event-data() -> ()  [unwired: 1 in, 3 out]
          }
          event Timeout {
            n67 = event-data() -> ()  [unwired: 1 in, 3 out]
          }
        }
      }
      n68 = while {
        shift-right: [w143] -> _
        shift-left: _ -> [w144]
        shift-right: [w142] -> _
        shift-left: _ -> [w145]
        tunnel: w116 -> [w140]
        tunnel: w115 -> [w141]
        tunnel: w107 -> [w133]
        tunnel: w106 -> [w132]
        shift-right: [w131] -> _
        shift-left: _ -> [w129]
        shift-right: [w130] -> _
        shift-left: _ -> [w128]
        shift-right: [w126] -> _
        shift-left: w105 -> [w122]
        shift-right: [w121] -> _
        shift-left: w104 -> [w120]
        stop <- w146 stop-if-true
        # "Elements in queue?"
        n69 = Get Queue Status(queue=w133, error in (no error)=w132) -> (queue out=w135:refnum<queue>, error out=w134:errorcluster, # elements in queue=w136:i32)  [unwired: 1 in, 5 out]
        n70 = Get Queue Status(queue=w140, error in (no error)=w141) -> (queue out=w138:refnum<queue>, error out=w137:errorcluster, # elements in queue=w139:i32)  [unwired: 1 in, 5 out]
        n71 = Greater Than 0?(x=w136) -> (x > 0?=w124:bool)
        n72 = Greater Than 0?(x=w139) -> (x > 0?=w123:bool)
        n73 = case shown="True" w124 {
          tunnel: w129 -> [w148 w169]
          tunnel: w128 -> [w149 w154]
          tunnel: [w149 w168] -> w130
          tunnel: [w148 w167] -> w131
          tunnel: w135 -> [_ w166]
          tunnel: w134 -> [_ w165]
          tunnel: "Save data" -> [_ w164]
          tunnel: [w147 w163] -> w126
          tunnel: w122 -> [w147 _]
          frame False {
          }
          frame True {
            (unwired) 1
            n74 = Flush Queue(queue=w166, error in (no error)=w165) -> (remaining elements=w153:T10)  [unwired: 2 out]
            n75 = for {
              tunnel: w153 -> [w181] mode=indexing
              shift-right: [w179] -> w150
              shift-left: _ -> [w178]
              shift-right: [w175] -> w152
              shift-left: _ -> [w174]
              shift-right: [w173] -> w151
              shift-left: _ -> [w172]
              i -> [w171]
              n76 = Unbundle(w181) -> ("Value:"=w180:dbl[], "Time:"=w177:string[], "Status:"=w176:string[])
              n77 = Greater Than 0?(x=w171) -> (x > 0?=w170:bool)
              n78 = case shown="False" w170 {
                tunnel: w180 -> [w184 w193]
                tunnel: [w184 w192] -> w179
                tunnel: w178 -> [_ w191]
                tunnel: w177 -> [w183 w190]
                tunnel: w176 -> [w182 w189]
                tunnel: [w183 w188] -> w175
                tunnel: w174 -> [_ w187]
                tunnel: [w182 w186] -> w173
                tunnel: w172 -> [_ w185]
                frame False {
                }
                frame True {
                  n79 = Build Array (concatenate)(w191, w193) -> (w192:dbl[])
                  n80 = Build Array (concatenate)(w190, w187) -> (w188:string[])
                  n81 = Build Array (concatenate)(w189, w185) -> (w186:string[])
                }
              }
            }
            n82 = for {
              tunnel: w152 -> [w216] mode=indexing
              tunnel: [w217] -> w160 mode=indexing
              # "Convert to timestamp"
              n83 = xnode "Match Regular Expression"("input string"=w216, "regular expression"="/") -> ("after match"=w215:string)  [unwired: 4 in, 4 out]
              n84 = Scan From String(format string="%<%H:%M:%S%3u>T", input string=w215) -> (output 1=w217:timestamp)  [unwired: 3 in, 3 out]
            }
            n85 = Build Array(w152, w151) -> (w155:string[][])
            n86 = Build Array (concatenate)(w154, w150) -> (w158:dbl[])
            n87 = local read "First Data point"() -> (w161:bool)
            n88 = case shown="True" w161 {
              tunnel: w160 -> [w201 w209]
              tunnel: [w199 w208] -> w156
              frame False {
                n89 = local read "Timestamp offset"() -> (w200:dbl)
                n90 = Add(x=w201, y=w200) -> (x+y=w199:timestamp[])
              }
              frame True {
                n91 = local write "First Data point"(FALSE) -> ()
                n92 = Get Date/Time In Seconds() -> (seconds since 1Jan1904=w212:timestamp)
                n93 = Index Array(array=w209, index=0) -> (element=w211:timestamp)
                n94 = Subtract(x=w212, y=w211) -> (x-y=w204:dbl)
                n95 = local write "Timestamp offset"(w204) -> ()
                n96 = Add(x=w209, y=w204) -> (x+y=w208:timestamp[])
                n97 = local read "tdms error"() -> (w206:errorcluster)
                n98 = local read "tdms file"() -> (w207:refnum<k34>)
                n99 = TDMS Set Properties(5:w204, 7:"Time offset" ("property names"), 8:w206, 11:w207) -> (0:w202:errorcluster, 3:w203:refnum<k34>)  [unwired: 2 in, 2 out]
                n100 = local write "tdms error"(w202) -> ()
                n101 = local write "tdms file"(w203) -> ()
              }
            }
            n102 = Build Array (concatenate)(w169, w156) -> (w157:timestamp[])
            n103 = case shown="True" "Reset graph 2" {
              tunnel: w156 -> [_ w198]
              tunnel: w150 -> [_ w197]
              tunnel: [w195 w198] -> w167
              tunnel: [w194 w197] -> w168
              tunnel: w158 -> [w194 _]
              tunnel: w157 -> [w195 _]
              frame False {
              }
              frame True {
                # "reset graph data?"
                n104 = local write "Reset graph 2"(FALSE) -> ()
              }
            }
            n105 = Bundle("Value:"=w150, w156, w155) -> (w163:cluster{"Value:":dbl[], timestamp[], string[][]})  [unwired: 1 in]
            n106 = case shown="True" w164 {
              tunnel: w156 -> [_ w335]
              tunnel: w150 -> [_ w336]
              tunnel: w155 -> [_ w346]
              frame False {
              }
              frame True {
                w337 = "Meter 2"
                n107 = local read "tdms error"() -> (w342:errorcluster)
                n108 = local read "tdms file"() -> (w343:refnum<k34>)
                n109 = TDMS Write(0:w343, 5:w337, 7:"Power", 9:w336, 11:w342) -> (4:w348:refnum<k34>, 15:w347:errorcluster)  [unwired: 1 in, 2 out]
                n110 = TDMS Write(0:w348, 5:w337, 7:string[] ["Time_L ", "Status"], 9:w346, 11:w347) -> (4:w334:refnum<k34>, 15:w333:errorcluster)  [unwired: 1 in, 2 out]
                n111 = TDMS Write(0:w334, 5:w337, 7:"Time_LV", 9:w335, 11:w333) -> (4:w341:refnum<k34>, 15:w340:errorcluster)  [unwired: 1 in, 2 out]
                n112 = TDMS Flush(4:w340, 7:w341) -> (0:w338:errorcluster, 3:w339:refnum<k34>)
                n113 = local write "tdms error"(w338) -> ()
                n114 = local write "tdms file"(w339) -> ()
              }
            }
            n115 = Bundle(w167, "Value:"=w168) -> (→"Power meter 2":cluster{timestamp[], "Value:":dbl[]})  [unwired: 1 in]
          }
        }
        n116 = case shown="True" w123 {
          tunnel: w145 -> [w351 w372]
          tunnel: w144 -> [w352 w371]
          tunnel: [w352 w370] -> w143
          tunnel: [w351 w369] -> w142
          tunnel: w138 -> [_ w368]
          tunnel: w137 -> [_ w367]
          tunnel: "Save data" -> [_ w366]
          tunnel: [w350 w365] -> w121
          tunnel: w120 -> [w350 _]
          frame False {
          }
          frame True {
            (unwired) 1
            # "Save files"
            # "If the first data point, then record that time as the time offset"
            # "reset graph data?"
            # "dump elements. the for loop is in case multiple elements were queued. Doubt this will happen"
            n117 = Flush Queue(queue=w368, error in (no error)=w367) -> (remaining elements=w353:T10)  [unwired: 2 out]
            n118 = for {
              tunnel: w353 -> [w540] mode=indexing
              shift-right: [w538] -> w364
              shift-left: _ -> [w537]
              shift-right: [w534] -> w363
              shift-left: _ -> [w533]
              shift-right: [w532] -> w362
              shift-left: _ -> [w531]
              i -> [w530]
              n119 = Unbundle(w540) -> ("Value:"=w539:dbl[], "Time:"=w536:string[], "Status:"=w535:string[])
              n120 = Greater Than 0?(x=w530) -> (x > 0?=w529:bool)
              n121 = case shown="False" w529 {
                tunnel: w539 -> [w543 w552]
                tunnel: [w543 w551] -> w538
                tunnel: w537 -> [_ w550]
                tunnel: w536 -> [w542 w549]
                tunnel: w535 -> [w541 w548]
                tunnel: [w542 w547] -> w534
                tunnel: w533 -> [_ w546]
                tunnel: [w541 w545] -> w532
                tunnel: w531 -> [_ w544]
                frame False {
                }
                frame True {
                  n122 = Build Array (concatenate)(w550, w552) -> (w551:dbl[])
                  n123 = Build Array (concatenate)(w549, w546) -> (w547:string[])
                  n124 = Build Array (concatenate)(w548, w544) -> (w545:string[])
                }
              }
            }
            n125 = for {
              tunnel: w363 -> [w395] mode=indexing
              tunnel: [w396] -> w359 mode=indexing
              # "Convert to timestamp"
              n126 = xnode "Match Regular Expression"("input string"=w395, "regular expression"="/") -> ("after match"=w393:string)  [unwired: 4 in, 4 out]
              n127 = Scan From String(format string="%<%H:%M:%S%3u>T", input string=w393) -> (output 1=w396:timestamp)  [unwired: 3 in, 3 out]
            }
            n128 = local read "First Data point"() -> (w360:bool)
            n129 = case shown="True" w360 {
              tunnel: w359 -> [w380 w388]
              tunnel: [w378 w387] -> w355
              frame False {
                n130 = local read "Timestamp offset"() -> (w379:dbl)
                n131 = Add(x=w380, y=w379) -> (x+y=w378:timestamp[])
              }
              frame True {
                n132 = local write "First Data point"(FALSE) -> ()
                n133 = local read "tdms error"() -> (w383:errorcluster)
                n134 = local read "tdms file"() -> (w385:refnum<k34>)
                n135 = Get Date/Time In Seconds() -> (seconds since 1Jan1904=w391:timestamp)
                n136 = Index Array(array=w388, index=0) -> (element=w390:timestamp)
                n137 = Subtract(x=w391, y=w390) -> (x-y=w384:dbl)
                "Timestamp offset" <- w384
                n138 = TDMS Set Properties(5:w384, 7:"Time offset" ("property names"), 8:w383, 11:w385) -> (0:w382:errorcluster, 3:w381:refnum<k34>)  [unwired: 2 in, 2 out]
                n139 = local write "tdms error"(w382) -> ()
                n140 = Add(x=w388, y=w384) -> (x+y=w387:timestamp[])
                n141 = local write "tdms file"(w381) -> ()
              }
            }
            n142 = Build Array (concatenate)(w371, w364) -> (w357:dbl[])
            n143 = Build Array (concatenate)(w372, w355) -> (w356:timestamp[])
            n144 = Build Array(w363, w362) -> (w354:string[][])
            n145 = case shown="True" w366 {
              tunnel: w355 -> [_ w512]
              tunnel: w364 -> [_ w513]
              tunnel: w354 -> [_ w525]
              frame False {
              }
              frame True {
                w514 = "Meter 1"
                n146 = local read "tdms error"() -> (w519:errorcluster)
                n147 = local read "tdms file"() -> (w520:refnum<k34>)
                n148 = TDMS Write(0:w520, 5:w514, 7:"Power", 9:w513, 11:w519) -> (4:w527:refnum<k34>, 15:w526:errorcluster)  [unwired: 1 in, 2 out]
                n149 = TDMS Write(0:w527, 5:w514, 7:string[] ["Time_L ", "Status"], 9:w525, 11:w526) -> (4:w523:refnum<k34>, 15:w522:errorcluster)  [unwired: 1 in, 2 out]
                n150 = TDMS Write(0:w523, 5:w514, 7:"Time_LV", 9:w512, 11:w522) -> (4:w518:refnum<k34>, 15:w517:errorcluster)  [unwired: 1 in, 2 out]
                n151 = TDMS Flush(4:w517, 7:w518) -> (0:w515:errorcluster, 3:w516:refnum<k34>)
                n152 = local write "tdms error"(w515) -> ()
                n153 = local write "tdms file"(w516) -> ()
              }
            }
            n154 = case shown="False" "Reset graph 1" {
              tunnel: w357 -> [w373 _]
              tunnel: w356 -> [w374 _]
              tunnel: w364 -> [_ w377]
              tunnel: w355 -> [_ w376]
              tunnel: [w373 w377] -> w370
              tunnel: [w374 w376] -> w369
              frame False {
              }
              frame True {
                n155 = local write "Reset graph 1"(FALSE) -> ()
              }
            }
            n156 = Bundle(w369, "Value:"=w370) -> (→"Power meter 1":cluster{timestamp[], "Value:":dbl[]})  [unwired: 1 in]
            n157 = Bundle("Value:"=w364, w355, w354) -> (w365:cluster{"Value:":dbl[], timestamp[], string[][]})  [unwired: 1 in]
          }
        }
        n158 = Or(x=w123, y=w124) -> (x .or. y?=w125:bool)
        n159 = case shown="True" w125 {
          tunnel: w121 -> [_ w555]
          tunnel: w126 -> [_ w553]
          frame False {
          }
          frame True {
            n160 = Bundle("output cluster 2"=w555, "output cluster 3"=w553) -> (→"output cluster":T1)  [unwired: 1 in]
          }
        }
        n161 = local read "Stop"() -> (w146:bool)
      }
      n162 = while {
        tunnel: w118 -> [w590]
        tunnel: w117 -> [_]
        tunnel: w114 -> [w597]
        tunnel: w119 -> [_]
        shift-right: [w593] -> _
        shift-left: _ -> [w594]
        stop <- w603 stop-if-true
        n163 = event shown="[1] \"Stop\": Value Change;  Panel Close" {
          selector: _ -> [_ _ _ _ _ _ _ _ _ _ _ _ _ _ _ _ _ _ _ _ _ _ _]
          dyn-events: _ -> [_ _ _ _ _ _ _ _ _ _ _ _ _ _ _ _ _ _ _ _ _ _ _]
          timeout: 10 -> [_ _ _ _ _ _ _ _ _ _ _ _ _ _ _ _ _ _ _ _ _ _ _]
          tunnel: [_ w627 _ _ _ _ _ _ _ _ _ _ _ _ _ _ _ _ _ _ _ _ _] -> w603
          tunnel: w590 -> [w616 w630 w640 w646 w664 w676 w688 w697 w722 w743 w757 _ w770 w784 w810 w823 w837 w844 w851 w859 w870 w878 _]
          tunnel: [w614 w625 w638 w645 w661 w668 w687 w699 w717 w738 w749 w762 w769 w774 w809 w814 w832 w839 w846 w854 w861 w880 w884] -> w593
          tunnel: "Gen'l Ops" -> [_ _ _ _ _ w673 w686 _ _ w742 w752 _ w767 w783 w811 _ w836 w843 w850 w858 w869 w883 _]
          tunnel: "All Handles" -> [_ w629 _ _ w656 _ w684 w689 w724 w741 w745 _ w768 w782 w812 w818 w835 w842 w849 w857 w868 w882 _]
          tunnel: "Read/Write" -> [_ _ _ _ _ _ _ _ _ _ _ _ _ _ _ _ _ _ _ _ w866 _ _]
          tunnel: "Dev Control" -> [_ _ _ _ _ _ _ _ _ _ _ _ w766 _ _ _ _ _ _ w853 _ _ _]
          tunnel: w597 -> [w618 w626 _ _ _ w670 _ w693 w721 _ w753 _ _ w780 w808 w821 _ _ _ _ _ _ _]
          tunnel: "scan again" -> [_ _ _ _ _ _ _ w698 _ _ _ _ _ _ _ _ _ _ _ _ _ _ _]
          tunnel: [_ w627 TRUE TRUE TRUE _ _ _ _ _ _ _ _ _ _ _ _ _ _ _ _ _ _] -> _
          tunnel: "Meas On" -> [_ _ _ _ _ _ _ _ w719 _ _ _ _ w778 w805 _ _ _ _ _ _ _ _]
          tunnel: w594 -> [w614 _ _ _ _ _ _ _ w717 _ _ w762 _ _ _ _ _ _ _ _ _ _ w884]
          event Timeout {
            # "Poll each Channel to handle user interactions"
            n164 = event-data() -> ()  [unwired: 2 out]
            n165 = for {
              tunnel: w618 -> [w624] mode=indexing
              tunnel: Channel_States."Poll" ("State") -> [w623]
              tunnel: w616 -> [w622]
              shift-right: [w619] -> _
              shift-left: errorcluster {"status"=FALSE, "code"=0, "source"=""} ("error out") -> [w620]
              n166 = call-by-ref "?"(reference=w624, "OphirLMMeasurementLib.ICoLMMeasurement"=w622, "State"=w623) -> ("error out"=w621:errorcluster)  [unwired: 9 in, 2 out]
              n167 = Merge Errors(w621, w620) -> (w619:errorcluster)
            }
          }
          event "Stop": Value Change; Panel Close {
            w627 = TRUE
            # "Close references to templates"
            # "Quit program"
            n168 = event-data() -> ()  [unwired: 3 out]
            n169 = for {
              tunnel: w630 -> [w632]
              tunnel: w629 -> [w634] mode=indexing
              tunnel: [w635] -> w628
              tunnel: w626 -> [w633]
              # "Stop streaming"
              # "Close all open handles"
              n170 = call "Stop All Channels streaming.vi"("Template Refs"=w633, "Handle"=w634, "LMMeasurementLib.ICoLMMeasurement"=w632) -> ("error out"=w631:errorcluster)
              n171 = invoke class="ICoLMMeasurement" method="Close"(reference=w632, error in=w631, "hDevice"=w634) -> (reference out=w635:refnum<k7>)  [unwired: 1 in, 3 out]
            }
            n172 = for {
              tunnel: w626 -> [w636] mode=indexing
              n173 = Close Reference(reference=w636) -> ()  [unwired: 1 in, 1 out]
            }
            n174 = Close Reference(reference=w628) -> (error out=w625:errorcluster)  [unwired: 1 in]
          }
          event "Get Lib Ver": Value Change {
            # "Get library verson from device"
            n175 = event-data() -> ()  [unwired: 2 out]
            n176 = invoke class="ICoLMMeasurement" method="GetVersion"(reference=w640) -> (error out=w638:errorcluster, "version"=→"LibVer":i32)  [unwired: 3 in, 2 out]
          }
          event "Get Driver Ver": Value Change {
            # "Get Driver Info from device"
            n177 = event-data() -> ()  [unwired: 2 out]
            n178 = invoke class="ICoLMMeasurement" method="GetDriverVersion"(reference=w646) -> (error out=w645:errorcluster, "info"=w644:string)  [unwired: 3 in, 2 out]
            n179 = Match Pattern(string=w644, regular expression="Version ") -> (after substring=→"DriverVer":string)  [unwired: 4 out]
          }
          event "Gen'l Ops.scanUSB", "scan again": Value Change {
            # "Look for all USB devices"
            n180 = event-data() -> ()  [unwired: 2 out]
            n181 = property on="Devices" class="MCListbox (strict)"() -> (error out=w655:errorcluster, "ItemNames"=w654:string[][])  [unwired: 2 in, 1 out]
            n182 = invoke class="ICoLMMeasurement" method="ScanUSB"(reference=w664, error in=w655) -> (error out=w661:errorcluster, "serialNumbers"=w663:variant)  [unwired: 2 in, 2 out]
            n183 = Index Array(array=w654, index (col) #1=0 ("disabled index (col)")) -> (element #1=w653:string[])  [unwired: 3 in, 1 out]
            n184 = Variant To Data(type=string[] [], Variant=w663) -> (data=w650:string[])  [unwired: 1 in, 1 out]
            n185 = call "Get Handles for Scan Devices.vi"("Old Device Names"=w653, "All Handles In"=w656, "New Device Names"=w650) -> ("All Handles Out"=w651:i32[], "# handles"=w657:i32)
            n186 = local write "All Handles"(w651) -> ()
            n187 = Initialize Array(FALSE, w657) -> (w658:bool[])
            n188 = local write "Meas On"(w658) -> ()
            n189 = Number To Decimal String(number=w651) -> (decimal integer string=w649:string[])  [unwired: 1 out]
            n190 = Build Array(w650, w649) -> (w648:string[][])
            n191 = Transpose 2D Array(2D array=w648) -> (transposed array=w647:string[][])
            n192 = property on="Devices" class="MCListbox (strict)"("ItemNames"=w647) -> ()  [unwired: 2 in, 2 out]
          }
          event "Gen'l Ops.Open": Value Change {
            # "When opening a device, send its\nhandle to each channel & store\nhandles in All Handles array"
            # "Open selected device"
            n193 = event-data() -> ()  [unwired: 2 out]
            n194 = property on="Devices" class="MCListbox (strict)"() -> ("ItemNames"=w674:string[][])  [unwired: 2 in, 2 out]
            n195 = Unbundle By Name(w673) -> ("Devices"=w672:i32)
            n196 = Index Array(array=w674, index (row)=w672, index (col)=0 ("disabled index (col)")) -> (element=w675:string)
            n197 = invoke class="ICoLMMeasurement" method="OpenUSBDevice"(reference=w676, "serialNumber"=w675) -> (reference out=w669:refnum<k7>, error out=w668:errorcluster, "hDevice"=w671:i32)  [unwired: 3 in, 2 out]
            n198 = control-ref of="Devices"() -> (w666:refnum<vi>)
            n199 = control-ref of="All Handles"() -> (w665:refnum<vi>)
            n200 = call "Set Handle on Open.vi"("error in"=w668, "All Handles ref"=w665, "hDevice"=w671, "Selected Device"=w672, "Ch refs"=w670, "OphirLMMeasurementLib.ICoLMMeasurement"=w669, "Devices List box ref"=w666) -> ()  [unwired: 3 out]
          }
          event "Gen'l Ops.Close": Value Change {
            # "Close selected device"
            n201 = event-data() -> ()  [unwired: 2 out]
            n202 = Unbundle By Name(w686) -> ("Devices"=w680:i32)
            n203 = Index Array(array=w684, index=w680) -> (element=w685:i32)
            n204 = Replace Array Subset(array=w684, new element=0 ("new element/subarray"), index=w680) -> (w683:i32[])
            n205 = invoke class="ICoLMMeasurement" method="Close"(reference=w688, "hDevice"=w685) -> (error out=w687:errorcluster)  [unwired: 2 in, 3 out]
            n206 = local write "All Handles"(w683) -> ()
            n207 = property on="Devices" class="MCListbox (strict)"() -> ("ItemNames"=w682:string[][])  [unwired: 2 in, 2 out]
            n208 = Replace Array Subset(array=w682, new element="0" ("new element/subarray"), index (row)=w680, index (col)=1 ("new element/subarray")) -> (w681:string[][])
            n209 = property on="Devices" class="MCListbox (strict)"("ItemNames"=w681) -> ()  [unwired: 2 in, 2 out]
          }
          event "Gen'l Ops.ResetAll": Value Change {
            # "This is an artificial method for generating an\nevent so the program will rescan the USB\nport after all devices are closed"
            # "Close all devices"
            n210 = event-data() -> ()  [unwired: 2 out]
            n211 = for {
              tunnel: w689 -> [w703] mode=indexing
              shift-right: [w704] -> w696
              shift-left: w697 -> [w705]
              tunnel: FALSE -> [w702]
              tunnel: Channel_States."Measure" ("State") -> [w701]
              tunnel: w693 -> [w700]
              # "For each device"
              n212 = for {
                shift-right: [w706] -> w704
                shift-left: w705 -> [w706]
                tunnel: w703 -> [w710]
                tunnel: w702 -> [w709]
                tunnel: w701 -> [w708]
                tunnel: w700 -> [w707] mode=indexing
                # "Turn off\nMeasure-\nments"
                # "For each channel"
                n213 = call-by-ref "?"(reference=w707, "Set Meas"=w709, "OphirLMMeasurementLib.ICoLMMeasurement"=w706, "Handle in"=w710, "State"=w708) -> ()  [unwired: 7 in, 3 out]
              }
            }
            n214 = Not(x=w698) -> ()  [unwired: 1 out]
            n215 = Array Size(array=w689) -> (size(s)=w690:i32)
            n216 = invoke class="ICoLMMeasurement" method="ResetAllDevices"(reference=w696) -> (error out=w699:errorcluster)  [unwired: 2 in, 2 out]
            n217 = Initialize Array(0 ("new element/subarray"), w690) -> (w692:i32[])
            n218 = local write "All Handles"(w692) -> ()
          }
          event "Gen'l Ops.Devices": Value Change {
            # "Update Handle to each Channel\n(this will also activate chs 2,3,4 if device\nis Pulsar)"
            # "Device changed, so update handle"
            n219 = event-data() -> ("NewVal"=w714:i32)  [unwired: 1 out]
            n220 = Index Array(array=w724, index=w714) -> (element=w711:i32)
            n221 = Number To Decimal String(number=w711) -> (decimal integer string=w712:string)  [unwired: 1 out]
            n222 = property on="Devices" class="MCListbox (strict)"() -> ("ItemNames"=w716:string[][])  [unwired: 2 in, 2 out]
            n223 = Replace Array Subset(array=w716, new element=w712, index (row)=w714, index (col)=1 ("disabled index (col)")) -> (w715:string[][])
            n224 = Index Array(array=w719, index=w714) -> (element=w718:bool)
            n225 = property on="Devices" class="MCListbox (strict)"("ItemNames"=w715) -> ()  [unwired: 2 in, 2 out]
            n226 = for {
              tunnel: w711 -> [w732]
              tunnel: Channel_States."Set Handle" ("State") -> [w731]
              tunnel: w721 -> [w730] mode=indexing
              tunnel: w722 -> [w727]
              tunnel: Channel_States."Measure" ("State") -> [w726]
              tunnel: w718 -> [w725]
              n227 = call-by-ref "?"(reference=w730, "OphirLMMeasurementLib.ICoLMMeasurement"=w727, "Handle in"=w732, "State"=w731) -> (reference out=w729:refnum<vi>, error out=w728:errorcluster)  [unwired: 8 in, 1 out]
              n228 = call-by-ref "?"(reference=w729, error in=w728, "Set Meas"=w725, "OphirLMMeasurementLib.ICoLMMeasurement"=w727, "State"=w726) -> ()  [unwired: 7 in, 3 out]
            }
          }
          event "Dev Control.UpdateInfo": Value Change {
            w734 = " - " ("string")
            n229 = event-data() -> ()  [unwired: 6 out]
            n230 = Unbundle By Name(w742) -> ("Devices"=w740:i32)
            n231 = Index Array(array=w741, index=w740) -> (element=w739:i32)
            n232 = invoke class="ICoLMMeasurement" method="GetDeviceInfo"(reference=w743, "hDevice"=w739) -> (error out=w738:errorcluster, "deviceName"=w737:string, "romVersion"=w736:string, "serialNumber"=w735:string)  [unwired: 5 in, 3 out]
            n233 = Concatenate Strings(w737, w734, w736, w734, w735) -> (→"Device Name":string)
          }
          event "Dev Control.ResetDev": Value Change {
            n234 = event-data() -> ()  [unwired: 2 out]
            n235 = Unbundle By Name(w752) -> ("Devices"=w744:i32)
            n236 = Index Array(array=w745, index=w744) -> (element=w748:i32)
            n237 = for {
              shift-right: [w758] -> w756
              shift-left: w757 -> [w758]
              tunnel: FALSE -> [w761]
              tunnel: Channel_States."Measure" ("State") -> [w760]
              tunnel: w753 -> [w759] mode=indexing
              # "Turn off\nMeasure-\nments"
              # "For each channel"
              n238 = call-by-ref "?"(reference=w759, "Set Meas"=w761, "OphirLMMeasurementLib.ICoLMMeasurement"=w758, "State"=w760) -> ()  [unwired: 8 in, 3 out]
            }
            n239 = invoke class="ICoLMMeasurement" method="ResetDevice"(reference=w756, "hDevice"=w748) -> (reference out=w751:refnum<k7>, error out=w750:errorcluster)  [unwired: 2 in, 2 out]
            n240 = Replace Array Subset(array=w745, new element=0 ("new element/subarray"), index=w744) -> (w746:i32[])
            n241 = local write "All Handles"(w746) -> ()
            n242 = invoke class="ICoLMMeasurement" method="Close"(reference=w751, error in=w750, "hDevice"=w748) -> (error out=w749:errorcluster)  [unwired: 1 in, 3 out]
          }
          event "Dev Control.ConfigCh", "Dev Control.Stream Modes:", "Dev Control.Value", "Dev Control.ExtTrig Window": Value Change {
            # "Don't do anything- Event loops need to handle changes of items changed\neven if they don't need to do anything with that change or the change won't\nbe used on the next iteration of the loop"
            n243 = event-data() -> ()  [unwired: 2 out]
          }
          event "Dev Control.SetConfig": Value Change {
            # "Sets the Channel, Stream Mode and Stream Mode Value for the current device"
            n244 = event-data() -> ()  [unwired: 2 out]
            n245 = Unbundle By Name(w767) -> ("Devices"=w771:i32)
            n246 = Index Array(array=w768, index=w771) -> (element=w772:i32)
            n247 = Unbundle By Name(w766) -> ("ConfigCh"=w765:i32, "Stream Modes:"=w764:i32, "Value"=w763:i32)
            n248 = invoke class="ICoLMMeasurement" method="ConfigureStreamMode"(reference=w770, "hDevice"=w772, "channel"=w765, "mode"=w764, "nValue"=w763) -> (error out=w769:errorcluster)  [unwired: 2 in, 6 out]
          }
          event "Dev Control.StartStream": Value Change {
            # "Start stream for all channels"
            n249 = event-data() -> ()  [unwired: 2 out]
            n250 = Unbundle By Name(w783) -> ("Devices"=w777:i32)
            n251 = Index Array(array=w782, index=w777) -> (element=w781:i32)
            n252 = for {
              tunnel: w784 -> [w792]
              tunnel: w781 -> [w788]
              tunnel: w780 -> [w787] mode=indexing
              tunnel: Channel_States."Measure" ("State") -> [w795]
              shift-right: [w793] -> w774
              shift-left: errorcluster {"status"=FALSE, "code"=0, "source"=""} ("error out") -> [w789]
              i -> [w786]
              n253 = invoke class="ICoLMMeasurement" method="IsSensorExists"(reference=w792, error in=w789, "hDevice"=w788, "channel"=w786) -> (reference out=w791:refnum<k7>, error out=w790:errorcluster, "exists"=w785:bool)  [unwired: 2 in, 3 out]
              n254 = case shown="True" w785 {
                tunnel: w786 -> [_ w803]
                tunnel: [w797 w802] -> w794
                tunnel: [w796 w801] -> w793
                tunnel: w791 -> [w797 w800]
                tunnel: w790 -> [w796 w799]
                tunnel: w788 -> [_ w798]
                frame False {
                  # "Sensor doesn't exist, so skip"
                }
                frame True {
                  n255 = invoke class="ICoLMMeasurement" method="StartStream"(reference=w800, error in=w799, "hDevice"=w798, "channel"=w803) -> (reference out=w802:refnum<k7>, error out=w801:errorcluster)  [unwired: 1 in, 3 out]
                }
              }
              n256 = call-by-ref "?"(reference=w787, "Set Meas"=w785, "OphirLMMeasurementLib.ICoLMMeasurement"=w794, "State"=w795) -> ()  [unwired: 8 in, 3 out]
            }
            n257 = Replace Array Subset(array=w778, new element=TRUE ("new element/subarray"), index=w777) -> (w775:bool[])
            n258 = local write "Meas On"(w775) -> ()
          }
          event "Dev Control.StopStream": Value Change {
            # "Stop stream for current channels"
            n259 = event-data() -> ()  [unwired: 2 out]
            n260 = Unbundle By Name(w811) -> ("Devices"=w813:i32)
            n261 = Index Array(array=w812, index=w813) -> (element=w804:i32)
            n262 = call "Stop All Channels streaming.vi"("Template Refs"=w808, "Handle"=w804, "LMMeasurementLib.ICoLMMeasurement"=w810) -> ("error out"=w809:errorcluster)
            n263 = Replace Array Subset(array=w805, new element=FALSE ("new element/subarray"), index=w804) -> (w806:bool[])
            n264 = local write "Meas On"(w806) -> ()
          }
          event "Dev Control.StopAll": Value Change {
            n265 = event-data() -> ()  [unwired: 2 out]
            n266 = Array Size(array=w818) -> (size(s)=w817:i32)
            n267 = Initialize Array(FALSE, w817) -> (w816:bool[])
            n268 = local write "Meas On"(w816) -> ()
            n269 = invoke class="ICoLMMeasurement" method="StopAllStreams"(reference=w823) -> (reference out=w820:refnum<k7>, error out=w814:errorcluster)  [unwired: 2 in, 1 out]
            n270 = for {
              tunnel: Channel_States."Measure" ("State") -> [w827]
              tunnel: w821 -> [w826] mode=indexing
              tunnel: w820 -> [w825]
              tunnel: FALSE -> [w824]
              # "Tells Channel Vis to stop measuring."
              n271 = call-by-ref "?"(reference=w826, "Set Meas"=w824, "OphirLMMeasurementLib.ICoLMMeasurement"=w825, "State"=w827) -> ()  [unwired: 8 in, 3 out]
            }
          }
          event "Dev Control.GetModes": Value Change {
            # "Gets External Trigger Modes from device and displays in externTrigModes"
            n272 = event-data() -> ()  [unwired: 2 out]
            n273 = Unbundle By Name(w836) -> ("Devices"=w834:i32)
            n274 = Index Array(array=w835, index=w834) -> (element=w833:i32)
            n275 = invoke class="ICoLMMeasurement" method="GetExtTrigModes"(reference=w837, "hDevice"=w833) -> (error out=w832:errorcluster, "index"=w829:i32, "options"=w830:variant)  [unwired: 4 in, 3 out]
            n276 = Variant To Data(type=string[] [], Variant=w830) -> (data=w828:string[])  [unwired: 1 in, 1 out]
            n277 = property on="externTrigModes" class="Ring (strict)"("Value"=w829, "Strings []"=w828) -> ()  [unwired: 2 in, 2 out]
          }
          event "Dev Control.externTrigModes": Value Change {
            # "Sets External Trigger Mode"
            n278 = event-data() -> ("NewVal"=w838:i32)  [unwired: 1 out]
            n279 = Unbundle By Name(w843) -> ("Devices"=w841:i32)
            n280 = Index Array(array=w842, index=w841) -> (element=w840:i32)
            n281 = invoke class="ICoLMMeasurement" method="SetExtTrigMode"(reference=w844, "hDevice"=w840, "index"=w838) -> (error out=w839:errorcluster)  [unwired: 2 in, 4 out]
          }
          event "Dev Control.GetWindow": Value Change {
            # "Gets External Trigger Window time from device and displays in extTrig Window"
            n282 = event-data() -> ()  [unwired: 2 out]
            n283 = Unbundle By Name(w850) -> ("Devices"=w848:i32)
            n284 = Index Array(array=w849, index=w848) -> (element=w847:i32)
            n285 = invoke class="ICoLMMeasurement" method="GetExtTrigWindowTime"(reference=w851, "hDevice"=w847) -> (error out=w846:errorcluster, "extTrigWindow"=w845:i32)  [unwired: 3 in, 3 out]
            n286 = property on="ExtTrig Window" class="DigNum (strict)"("Value"=w845) -> ()  [unwired: 2 in, 2 out]
          }
          event "Dev Control.Modify": Value Change {
            # "Set external trigger window time"
            n287 = event-data() -> ()  [unwired: 2 out]
            n288 = Unbundle By Name(w858) -> ("Devices"=w856:i32)
            n289 = Unbundle By Name(w853) -> ("ExtTrig Window"=w852:i32)
            n290 = Index Array(array=w857, index=w856) -> (element=w855:i32)
            n291 = invoke class="ICoLMMeasurement" method="SetExtTrigWindowTime"(reference=w859, "hDevice"=w855, "extTrigWindowTime"=w852) -> (error out=w854:errorcluster)  [unwired: 2 in, 4 out]
          }
          event "Read/Write.Write": Value Change {
            # "Writes the value in the Writestr control to the device.  If AutoRead = True, then it also reads from the device and displays the result in ReadStr"
            n292 = event-data() -> ()  [unwired: 2 out]
            n293 = Unbundle By Name(w869) -> ("Devices"=w867:i32)
            n294 = Unbundle By Name(w866) -> ("WriteStr"=w865:string, "AutoRead"=w864:bool)
            n295 = Index Array(array=w868, index=w867) -> (element=w860:i32)
            n296 = invoke class="ICoLMMeasurement" method="Write"(reference=w870, "hDevice"=w860, "command"=w865) -> (reference out=w863:refnum<k7>, error out=w862:errorcluster)  [unwired: 2 in, 3 out]
            n297 = case shown="True" w864 {
              tunnel: w863 -> [_ w876]
              tunnel: w862 -> [w871 w875]
              tunnel: [w871 w873] -> w861
              tunnel: w860 -> [_ w874]
              frame False {
              }
              frame True {
                n298 = invoke class="ICoLMMeasurement" method="Read"(reference=w876, error in=w875, "hDevice"=w874) -> (error out=w873:errorcluster, "reply"=→"ReadStr":string)  [unwired: 2 in, 3 out]
              }
            }
          }
          event "Read/Write.Read": Value Change {
            # "Reads from the device and displays the result in ReadStr"
            n299 = event-data() -> ()  [unwired: 2 out]
            n300 = Unbundle By Name(w883) -> ("Devices"=w881:i32)
            n301 = Index Array(array=w882, index=w881) -> (element=w879:i32)
            n302 = invoke class="ICoLMMeasurement" method="Read"(reference=w878, "hDevice"=w879) -> (error out=w880:errorcluster, "reply"=w877:string)  [unwired: 3 in, 3 out]
            n303 = local write "ReadStr"(w877) -> ()
          }
          event "Read/Write.AutoRead": Value Change {
            # "Don't do anything- Event loops need to handle changes of items changed\neven if they don't need to do anything with that change or the change won't\nbe used on the next iteration of the loop"
            n304 = event-data() -> ()  [unwired: 6 out]
          }
        }
        n305 = Unbundle By Name(w593) -> ("code"=w591:i32)
        n306 = Not Equal?(x=w594, y=w593) -> (x != y?=w592:bool)
        n307 = case shown="False" w592 {
          tunnel: w591 -> [w613 _]
          tunnel: w590 -> [w612 _]
          frame False {
            n308 = invoke class="ICoLMMeasurement" method="GetErrorFromCode"(reference=w612, "errorCode"=w613) -> ("errorString"=w605:string)  [unwired: 3 in, 4 out]
            "Last Error Code:" <- w605
            n309 = Equal?(x="No Error", y=w605) -> (x = y?=w606:bool)
            n310 = Empty String/Path?(string/path=w605) -> (empty?=w607:bool)
            n311 = Or(x=w606, y=w607) -> (x .or. y?=w608:bool)
            n312 = Select(t=u32 0, s=w608, f=u32 15667968) -> (s? t:f=w604:u32)
            n313 = property on="Last Error Code:" class="Str"("Text.FontColor"=w604) -> ()  [unwired: 2 in, 2 out]
          }
          frame True {
          }
        }
      }
    }
    frame #2 {
      # "try just using new val in event structure"
      # "Closes program if running\nas exe"
      n314 = property class="App"() -> ("App.Kind"=w930:T8)  [unwired: 2 in, 2 out]
      n315 = Equal?(x=w930, y=T8."Run Time System") -> (x = y?=w931:bool)
      n316 = Quit LabVIEW(quit? (T)=w931) -> ()
      n317 = Unregister For Events(event registration refnum=w922) -> ()  [unwired: 1 in, 1 out]
      n318 = Release Queue(queue=w921, error in (no error)=w920) -> ()  [unwired: 1 in, 3 out]
      n319 = Release Queue(queue=w919, error in (no error)=w918) -> ()  [unwired: 1 in, 3 out]
      n320 = Unregister For Events(event registration refnum=w923) -> ()  [unwired: 1 in, 1 out]
      n321 = local write "Stop"(FALSE ("stop")) -> ()
      n322 = TDMS Close(8:w927, 11:w926) -> (0:w928:errorcluster)  [unwired: 1 out]
      n323 = call <vilib>:"Simple Error Handler.vi"("error in (no error)"=w928) -> ()  [unwired: 4 in, 5 out]
      "First Data point" <- TRUE
    }
  }
